vi "Задание_АБ_добавляем_демодуляцию.vi"() -> ()   [LabVIEW 2017]
uses:
  <vilib>/Analysis/NI_AALBase.lvlib
panel:
  out "x*y":dbl[](array[numeric])
  out "Array":dbl[][](array[numeric])
  out "Модулирующий сигнал":dbl[](graph)
  out "Частотно модулированный цифровой сигнал":dbl[][](graph)
  in  "см. 1.2 Циклов в секунду":i32(slide) scale=4.0..50.0
  in  "Сколько битов брать":i32=4
  out "Радио сигнал с паузами":dbl[](graph)
  in  "Кол-во выборок":i32=400
  out "Массив с паузами":dbl[](array[numeric])
  in  "Количество бит":i32=8
  out "Вырезка из массива":dbl[](array[numeric])
  out "Биты на выходе 1":dbl[](array[numeric])
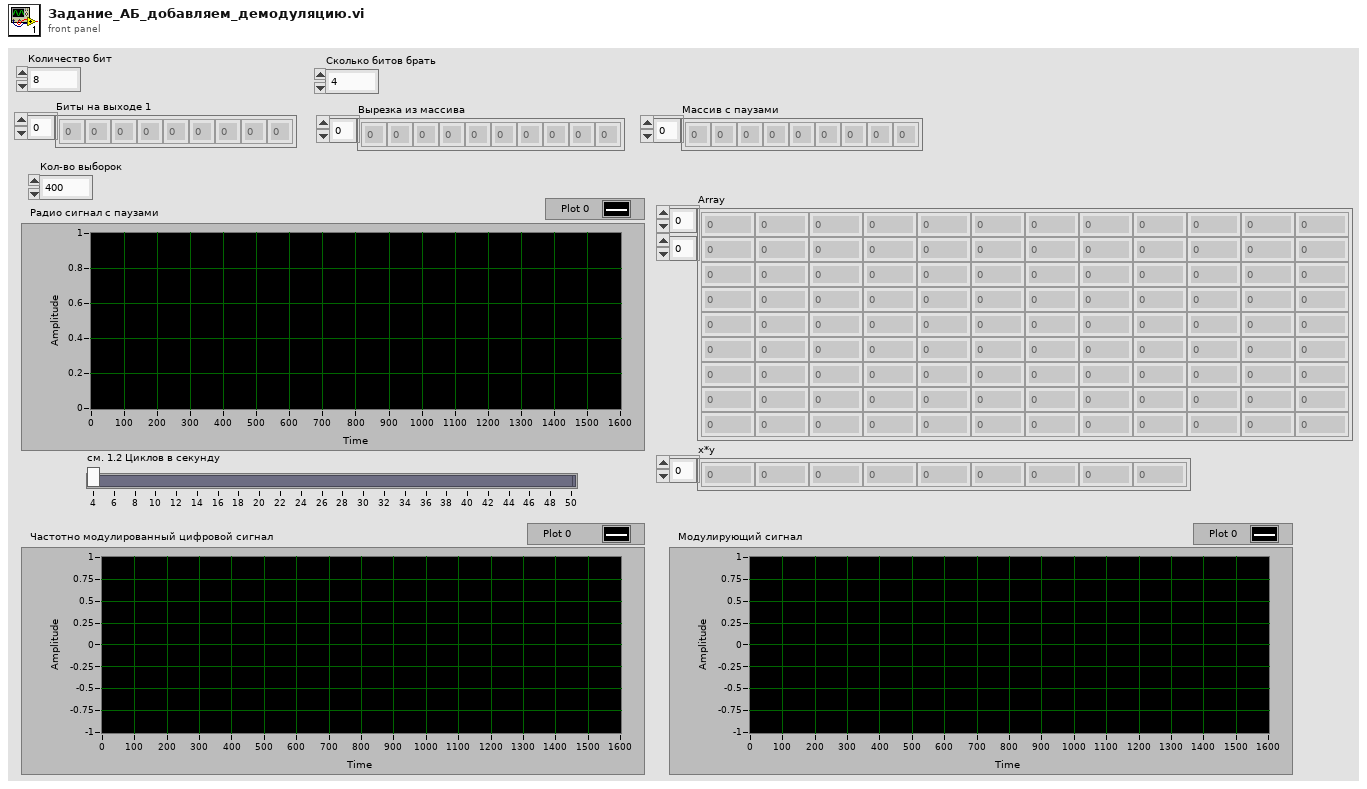
[diagram p1: front panel]
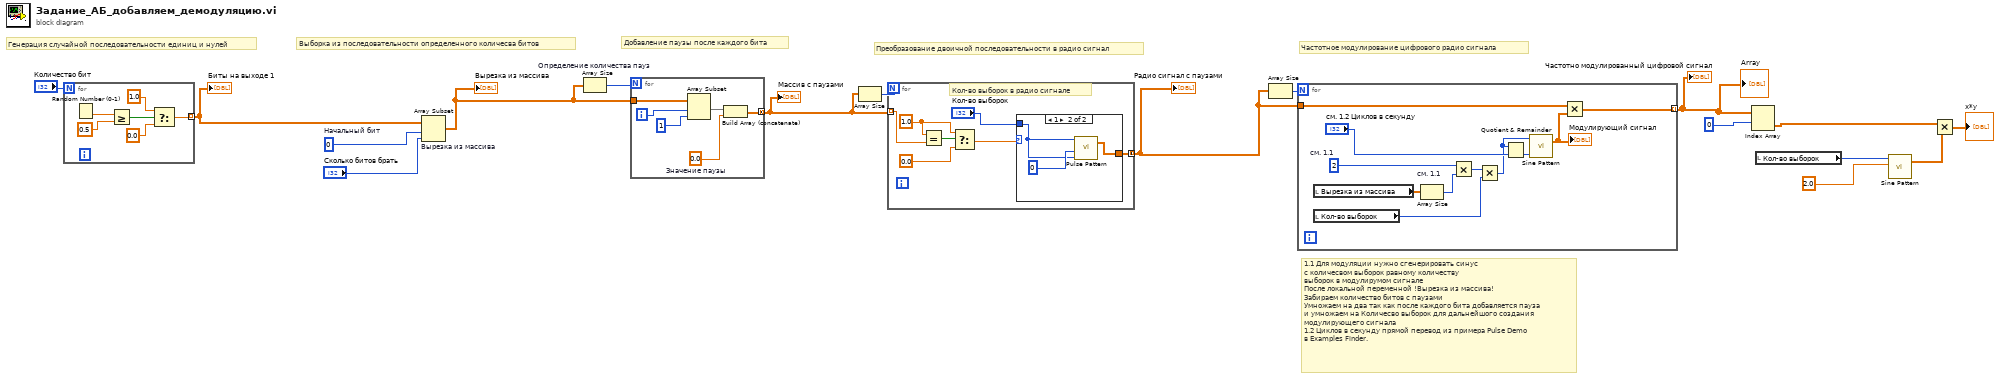
[diagram p0: block diagram]
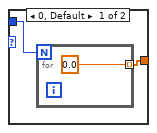
[diagram p2: hidden frame]
diagram:
  w16 = 0  # Начальный бит
  # "1.1 Для модуляции нужно сгенерировать синус \nс количесвом выборок равному количеству \nвыборок в модулирумом сигнале\nПосле локальной переменной !Вырезка из массива! \nЗабираем количество битов с паузами \nУмножаем на два так как после каждого бита добавляется пауза\nи умножаем на Количесво выборок для дальнейшого создания  \nмодулирующего сигнала\n1.2 Циклов в секунду прямой перевод из примера Pulse Demo \nв Examples Finder."
  # "Преобразование двоичной последовательности в радио сигнал"
  # "Частотное модулирование цифрового радио сигнала"
  # "Добавление паузы после каждого бита"
  # "Выборка из последовательности определенного количесва битов"
  # "Генерация случайной последовательности единиц и нулей"
  n1 = for {
    N: "Количество бит" -> [_]
    tunnel: [w18] -> w14 mode=indexing
    n2 = Random Number (0-1)() -> (number: 0 to 1=w23:dbl)
    n3 = Greater Or Equal?(x=w23, y=0.5) -> (x >= y?=w21:bool)
    n4 = Select(t=1.0, s=w21, f=0.0) -> (s? t:f=w18:dbl)
  }
  "Биты на выходе 1" <- w14
  n5 = Array Subset "Вырезка из массива"(array=w14, index=w16, length="Сколько битов брать") -> (w12:dbl[])
  "Вырезка из массива" <- w12
  n6 = Array Size "Определение количества пауз"(array=w12) -> (size(s)=w13:i32)
  n7 = for {
    N: w13 -> [_]
    tunnel: w12 -> [w26]
    tunnel: [w25] -> w9 mode=concatenating
    i -> [w24]
    w27 = 0.0  # Значение паузы
    n8 = Array Subset(array=w26, index=w24, length=1) -> (w28:dbl[])
    n9 = Build Array (concatenate)(w28, w27) -> (w25:dbl[])
  }
  "Массив с паузами" <- w9
  n10 = Array Size(array=w9) -> (size(s)=w10:i32)
  n11 = for {
    N: w10 -> [_]
    tunnel: w9 -> [w33] mode=indexing
    tunnel: [w31] -> w8 mode=concatenating
    w35 = 1.0
    # "Кол-во выборок в радио сигнале"
    n12 = Equal?(x=w35, y=w33) -> (x = y?=w36:bool)
    n13 = Select(t=w35, s=w36, f=0.0) -> (s? t:f=w32:dbl)
    n14 = case shown="1" w32 {
      tunnel: [w37 w41] -> w31
      tunnel: "Кол-во выборок" -> [w38 w40]
      frame 0, Default {
        n15 = for {
          N: w38 -> [_]
          tunnel: [0.0] -> w37 mode=indexing
        }
      }
      frame 1 {
        n16 = call <vilib>:"Pulse Pattern.vi"("width"=w40, "delay"=0, "samples"=w40) -> ("Pulse Pattern"=w41:dbl[])  [unwired: 1 in, 1 out]
      }
    }
  }
  "Радио сигнал с паузами" <- w8
  n17 = Array Size(array=w8) -> (size(s)=w11:i32)
  n18 = for {
    N: w11 -> [_]
    tunnel: w8 -> [w51]
    tunnel: [w50] -> w7 mode=indexing
    w46 = 2  # см. 1.1
    n19 = local read "Вырезка из массива"() -> (w48:dbl[])
    n20 = local read "Кол-во выборок"() -> (w44:i32)
    n21 = Array Size "см. 1.1"(array=w48) -> (size(s)=w47:i32)
    n22 = Multiply(x=w46, y=w47) -> (x*y=w45:i32)
    n23 = Multiply(x=w45, y=w44) -> (x*y=w43:i32)
    n24 = Quotient & Remainder(x=w43, y="см. 1.2 Циклов в секунду") -> (floor(x/y)=w53:i32)  [unwired: 1 out]
    n25 = call <vilib>:"Sine Pattern.vi"("cycles"=w53, "samples"=w43) -> ("Sinusoidal Pattern"=w49:dbl[])  [unwired: 2 in, 1 out]
    "Модулирующий сигнал" <- w49
    n26 = Multiply(x=w51, y=w49) -> (x*y=w50:dbl[])
  }
  "Частотно модулированный цифровой сигнал" <- w7
  "Array" <- w7
  n27 = Index Array(array=w7, index (row)=0) -> (element=w5:dbl[])  [unwired: 1 in]
  n28 = local read "Кол-во выборок"() -> (w4:i32)
  n29 = call <vilib>:"Sine Pattern.vi"("amplitude"=2.0, "samples"=w4) -> ("Sinusoidal Pattern"=w2:dbl[])  [unwired: 2 in, 1 out]
  n30 = Multiply(x=w5, y=w2) -> (x*y=→"x*y":dbl[])
